vi "pythonDeallocateArrayUINT16.vi"(1 "ptr":i64) -> ()   [LabVIEW 2017]
uses:
  dll/wormUtilities/x64/Release/wormUtilities.dll
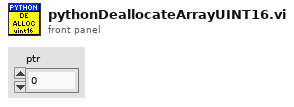
[diagram p1: front panel]
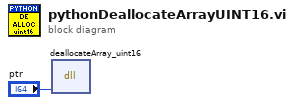
[diagram p0: block diagram]
diagram:
  n1 = dll-call lib="C:/Users/francesco/dev/pump-probe/dll/wormUtilities/x64/Release/wormUtilities.dll" fn="deallocateArray_uint16"("ptr"="ptr") -> ()  [unwired: 5 in, 2 out]
